vi "ARRAY3D.vi"() -> ()   [LabVIEW 2023]
doc: "This function sums each element in pages 0 through n-2 of an n page sized 3-D array and places the values in the corresponding element on page n-1. It is assumed that page n-1 is already allocated in the input array.\n\nFor information on the data types used for the DLL function, right-click on the Call Library Function node and choose Configure."
uses:
  CLF_Example.dll
panel:
  out "output":dbl[][][](array[numeric])
  in  "input":dbl[][][](array[numeric])=[[[0.0, 1.0], [2.0, 3.0], [4.0, 5.0], [6.0, 7.0]], [[0.0, 2.0], [4.0, 6.0], [8.0, 10.0], [12.0, 14.0]], [[0.0, 0.0], [0.0, 0.0], [0.0, 0.0], [0.0, 0.0]], [[0.0, 1.0], [2.0, 3.0], [4.0, 5.0], [6.0, 7.0]]]
  # "See the block diagram for more information."
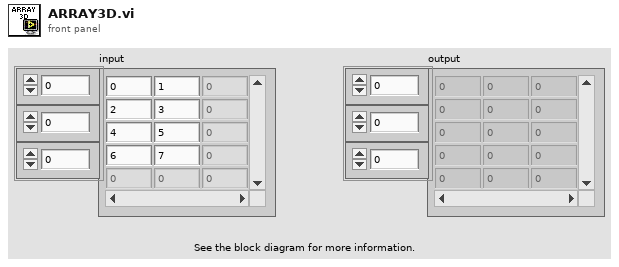
[diagram p1: front panel]
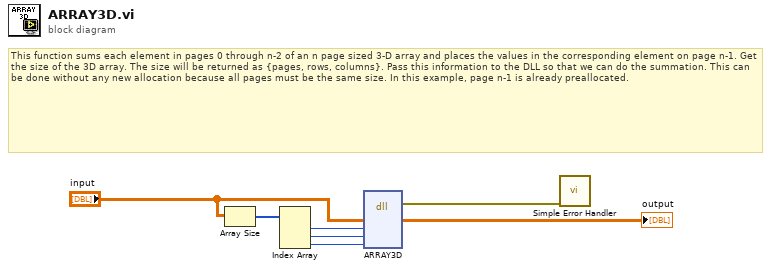
[diagram p0: block diagram]
diagram:
  # "This function sums each element in pages 0 through n-2 of an n page sized 3-D array and places the values in the corresponding element on page n-1. Get the size of the 3D array. The size will be returned as {pages, rows, columns}. Pass this information to the DLL so that we can do the summation. This can be done without any new allocation because all pages must be the same size. In this example, page n-1 is already preallocated."
  n1 = Array Size(array="input") -> (size(s)=w5:i32[])
  n2 = Index Array(array=w5) -> (element #1=w4:i32, element #2=w3:i32, element #3=w2:i32)  [unwired: 3 in]
  n3 = dll-call lib="c:/dev/_r/4/eng/lv-core/lvpostprocessingd/lv_mc_x86_64/dist_i386/examples/Connectivity/Libraries and Executables/DLL Calling VIs/CLF_Example**.*" fn="ARRAY3D"("array"="input", "array_length_page"=w4, "array_length_row"=w3, "array_length_col"=w2) -> (error out=w1:errorcluster, "array"=→"output":dbl[][][])  [unwired: 6 in, 2 out]
  n4 = call <vilib>:"Simple Error Handler.vi"("error in (no error)"=w1) -> ()  [unwired: 4 in, 5 out]
